vi "Swerve Motor Brushless BL v2.vi"(3 "Offset":dbl, 4 "Drive Commands":T2, 6 "Direction command (deg)":dbl, 7 "Speed command":dbl, 9 "Align 90":bool) -> (0 "Back Left Position":dbl, 1 "Back Left Current Angle":dbl, 2 "Back Left Velocity":dbl)   [LabVIEW 2020]
uses:
  <vilib>/Analysis/coordinate.llb/Angle Units.ctl
  <vilib>/Analysis/coordinate.llb/Angle Range (Degree).ctl
  <vilib>/Rock Robotics/WPI/ThirdParty/REV Robotics/REVLib/Typedef/Spark MAX Control Type.ctl
  <vilib>/Analysis/coordinate.llb/Wrap Angle (scalar).vi
  <vilib>/addons/control/pid/pid.llb/PID (DBL).vi
  <vilib>/Analysis/NI_AAL_Angle.lvlib
  <vilib>/addons/control/pid/NI_PID_pid.lvlib
panel:
  out "Encoder Count to Move":dbl
  out "Better Angle":dbl(knob)=41.7137932364482 scale=0.0..360.0
  out "Degres To Travel":dbl
  out "Position Closed Loop Plots":cluster{"Better Position":dbl, dbl}(graph)
  in  "PID gains":T1={"proportional gain (Kc)"=0.01, "integral time (Ti, min)"=0.0, "derivative time (Td, min)"=0.004} {"integral time (Ti, min)" format="%#_6f"; "derivative time (Td, min)" format="%#_6f"}
  in  "output range":cluster{"output high":dbl, "output low":dbl}={"output high"=0.4, "output low"=-0.4} {"output low" format="%.2f"; "output high" format="%.2f"}
  out "Flip motors?":bool
  out "Better Position":dbl
  # "VI inputs"
  # "Intermediate values"
  # "Click here to set min"
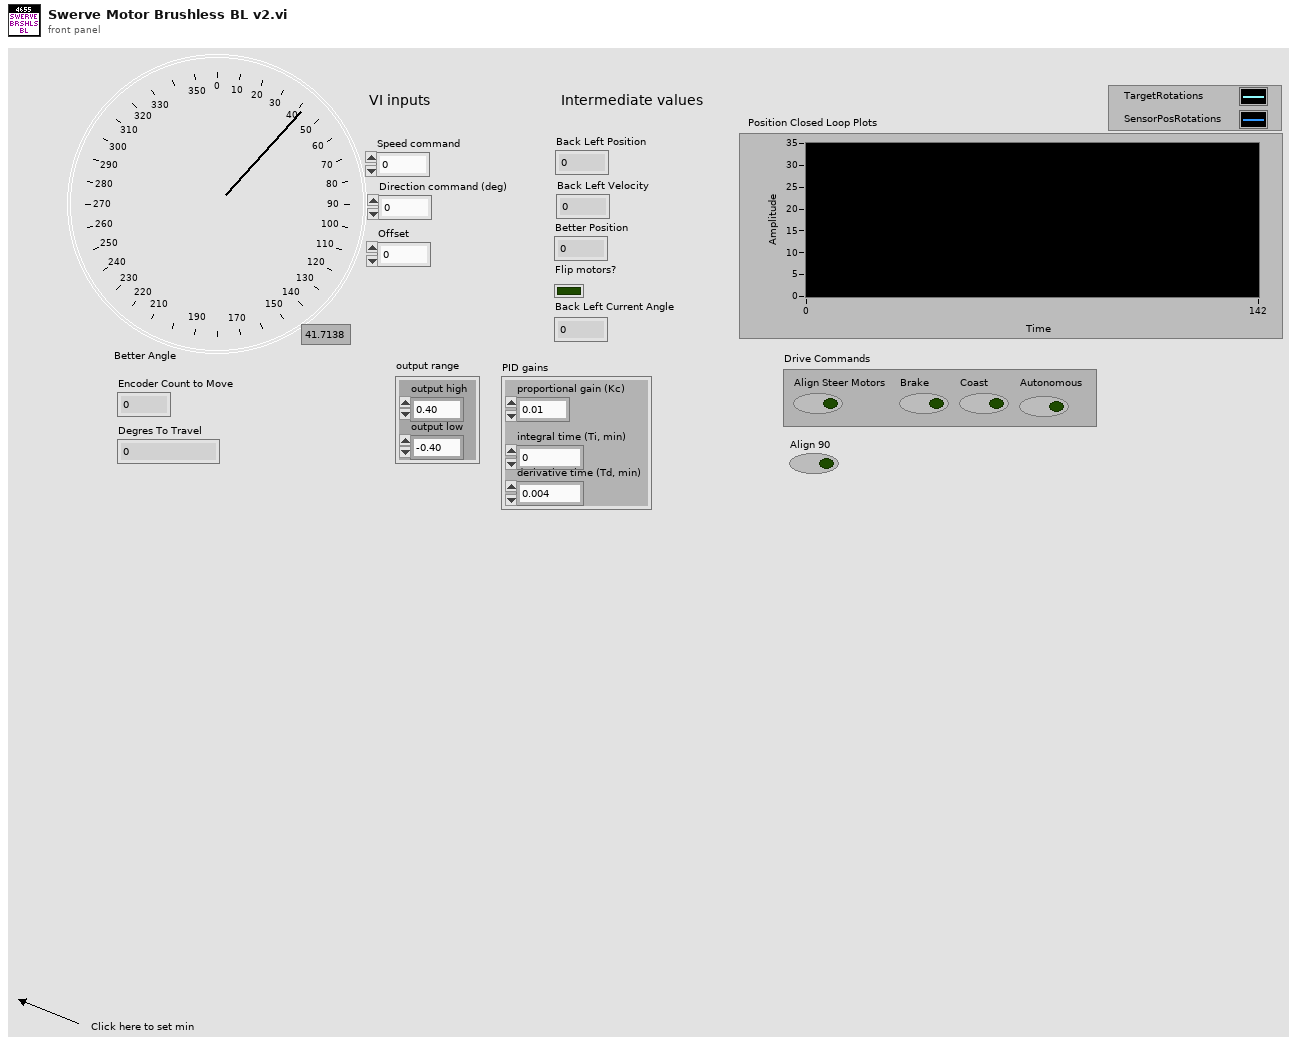
[diagram p1: front panel]
types:
  T1 = cluster{"proportional gain (Kc)":dbl, "integral time (Ti, min)":dbl, "derivative time (Td, min)":dbl}
  T2 = cluster{"Align Steer Motors":bool, "Brake":bool, "Coast":bool, "Autonomous":bool}
  T3 = typedef "NI_AAL_Angle.lvlib/Angle Range (Degree).ctl" = u16
  T4 = typedef "NI_AAL_Angle.lvlib/Angle Units.ctl" = i32
  T5 = typedef "WPI_MotorControlDeviceRef.ctl" = cluster{"DeviceStatus":errorcluster, "Type":T6, "PWM":cluster{"PWM Channel":T7, "DeadBand":T8}, "CAN":cluster{"Device Number":u8, "SetOutput VI Ref":variant, "GetOutput VI Ref":variant, "Enable VI Ref":variant, "Disable VI Ref":variant, "Data":variant}, "Invert":bool, "DIO PWM":cluster{"PWM \"Enable\" Channel":T7, "DIOChannel":T9, "PWM Rate":dbl}}
  T6 = typedef "WPI_MotorControlType.ctl" = enum16{"PWM", "CAN", "DIO PWM"}
  T7 = typedef "FPGA_DIOPWMChannel.ctl" = enum8{"PWM 0", "PWM 1", "PWM 2", "PWM 3", "PWM 4", "PWM 5", "PWM 6", "PWM 7", "PWM 8", "PWM 9", "PWM MXP 0", "PWM MXP 1", "PWM MXP 2", "PWM MXP 3", "PWM MXP 4", "PWM MXP 5", "PWM MXP 6", "PWM MXP 7", "PWM MXP 8", "PWM MXP 9", "Invalid"}
  T8 = typedef "WPI_PWMDeadband.ctl" = cluster{"Name":string, "maxPositivePwm":i32, "minPositivePwm":i32, "centerPwm":i32, "maxNegativePwm":i32, "minNegativePwm":i32, "angularRange":u16}
  T9 = typedef "FPGA_DIOChannel.ctl" = enum8{"DIO 0", "DIO 1", "DIO 2", "DIO 3", "DIO 4", "DIO 5", "DIO 6", "DIO 7", "DIO 8", "DIO 9", "DIO MXP 0", "DIO MXP 1", "DIO MXP 2", "DIO MXP 3", "DIO MXP 4", "DIO MXP 5", "DIO MXP 6", "DIO MXP 7", "DIO MXP 8", "DIO MXP 9", "DIO MXP 10", "DIO MXP 11", "DIO MXP 12", "DIO MXP 13", "DIO MXP 14", "DIO MXP 15", "SPI Port CS1", "SPI Port CS2", "SPI Port CS3", "SPI Port MISO", "SPI Port MOSI", "Invalid"}
  T10 = cluster{"process variable":dbl, "Degres To Travel":dbl}
  T11 = typedef "Spark MAX Control Type.ctl" = enum16{"Percent VBus", "Voltage", "Velocity", "Position", "Smart Motion", "Current", "Smart Velocity"}
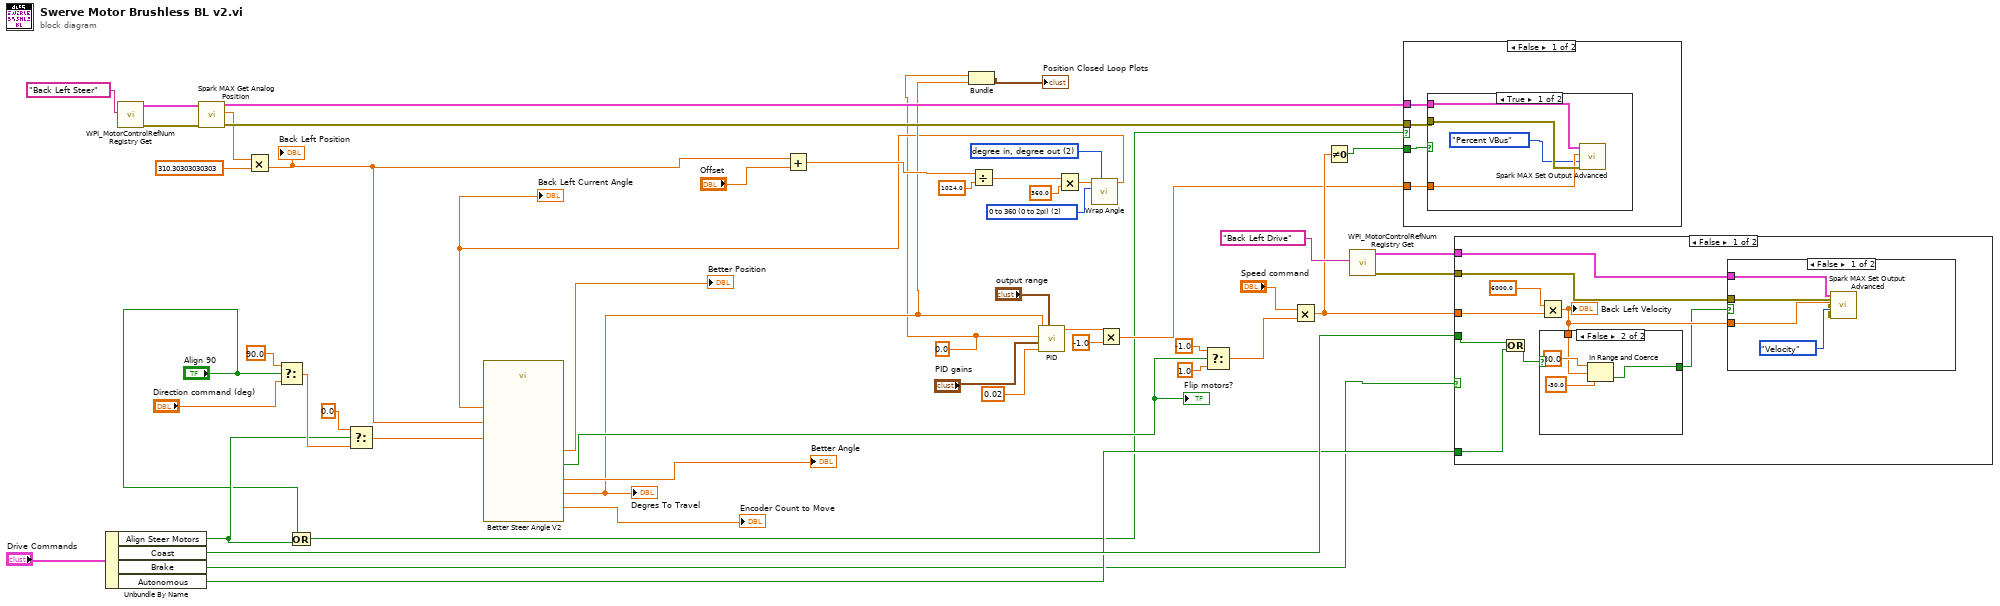
[diagram p0: block diagram]
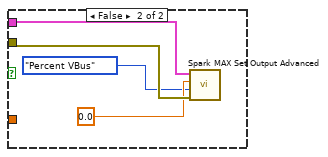
[diagram p2: hidden frame]
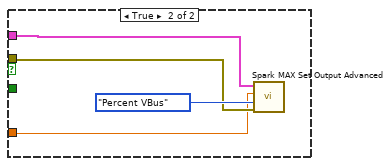
[diagram p3: hidden frame]
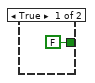
[diagram p4: hidden frame]
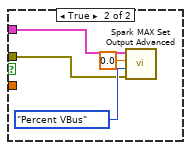
[diagram p5: hidden frame]
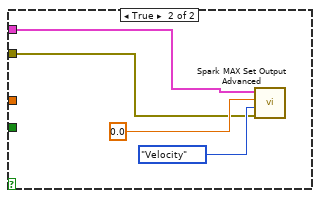
[diagram p6: hidden frame]
diagram:
  w2 = 0.0 ("process variable")
  w42 = T3 2 items=["none", "-180 to 180 (-pi to pi)", "0 to 360 (0 to 2pi)"] ("angle range")
  w43 = T4 2 items=["radian in, radian out", "radian in, degree out", "degree in, degree out", "degree in, radian out"] ("angle units")
  n1 = Unbundle By Name("Drive Commands") -> ("Align Steer Motors"=w10:bool, "Coast"=w38:bool, "Brake"=w36:bool, "Autonomous"=w37:bool)
  n2 = call <vilib>:"WPI_MotorControlRefNum Registry Get.vi"("refnum name"="Back Left Steer" ("Motor References")) -> ("error out"=w34:errorcluster, "RobotDriveDevRef"=w35:T5)  [unwired: 9 in]
  n3 = call <vilib>:"Spark MAX Get Analog Position.vi"("error in (no error)"=w34, "MotorControlDevRef in"=w35) -> ("error out"=w47:errorcluster, "Analog Position"=w18:dbl, "MotorControlDevRef out"=w20:T5)  [unwired: 6 in, 1 out]
  n4 = Multiply(x=w18, y=310.30303030303) -> (x*y=w6:dbl)
  "Back Left Position" <- w6
  n5 = Select(t=90.0, s="Align 90", f="Direction command (deg)") -> (s? t:f=w15:dbl)
  n6 = Or(x="Align 90", y=w10) -> (x .or. y?=w11:bool)
  n7 = Select(t=0.0, s=w10, f=w15) -> (s? t:f=w12:dbl)
  n8 = Add(x=w6, y="Offset") -> (x+y=w23:dbl)
  n9 = Divide(x=w23, y=1024.0 ("x")) -> (x/y=w41:dbl)
  n10 = Multiply(x=w41, y=360.0 ("x*y")) -> (x*y=w40:dbl)
  n11 = call-poly <vilib>:"Wrap Angle.vi"("angle units"=w43, "angle range"=w42, "angle in"=w40) -> ("angle out"=w3:dbl)  [unwired: 7 in, 1 out]
  "Back Left Current Angle" <- w3
  n12 = call "Better Steer Angle V2.vi"("Current Angle"=w3, "Current Position"=w6, "Set Point In"=w12) -> ("Better Angle"=→"Better Angle":dbl, "Better Position"=→"Better Position":dbl, "Encoder Count to Move"=→"Encoder Count to Move":dbl, "Flip motors?"=w46:bool, "Degres To Travel"=w4:dbl)
  "Flip motors?" <- w46
  "Degres To Travel" <- w4
  n13 = Bundle("process variable"=w2, "Degres To Travel"=w4) -> (→"Position Closed Loop Plots":T10)  [unwired: 1 in]
  n14 = call-poly <vilib>:"PID.vi"("output range"="output range", "dt (s)"=0.02, "PID gains"="PID gains", "process variable"=w2, "setpoint"=w4) -> ("output"=w22:dbl)  [unwired: 5 in, 1 out]
  n15 = Multiply(x=w22, y=-1.0) -> (x*y=w19:dbl)
  n16 = Select(t=-1.0, s=w46, f=1.0) -> (s? t:f=w49:dbl)
  n17 = Multiply(x="Speed command", y=w49) -> (x*y=w21:dbl)
  n18 = Not Equal To 0?(x=w21) -> (x != 0?=w1:bool)
  n19 = call <vilib>:"WPI_MotorControlRefNum Registry Get.vi"("refnum name"="Back Left Drive" ("Motor References")) -> ("error out"=w30:errorcluster, "RobotDriveDevRef"=w31:T5)  [unwired: 9 in]
  n20 = case shown="False" w11 {
    tunnel: w47 -> [w55 w66]
    tunnel: w1 -> [w54 _]
    tunnel: w20 -> [w53 w65]
    tunnel: w19 -> [w52 w64]
    frame False {
      n21 = case shown="True" w54 {
        tunnel: w53 -> [w59 w63]
        tunnel: w55 -> [w58 w62]
        tunnel: w52 -> [w57 _]
        frame True {
          n22 = call <vilib>:"Spark MAX Set Output Advanced.vi"("error in (no error)"=w58, "Control Mode"=Spark_MAX_Control_Type."Percent VBus", "Setpoint"=w57, "MotorControlDevRef"=w59) -> ()  [unwired: 6 in, 2 out]
        }
        frame False {
          n23 = call <vilib>:"Spark MAX Set Output Advanced.vi"("error in (no error)"=w62, "Control Mode"=Spark_MAX_Control_Type."Percent VBus", "Setpoint"=0.0 ("y"), "MotorControlDevRef"=w63) -> ()  [unwired: 6 in, 2 out]
        }
      }
    }
    frame True {
      n24 = call <vilib>:"Spark MAX Set Output Advanced.vi"("error in (no error)"=w66, "Control Mode"=Spark_MAX_Control_Type."Percent VBus", "Setpoint"=w64, "MotorControlDevRef"=w65) -> ()  [unwired: 6 in, 2 out]
    }
  }
  n25 = case shown="False" w36 {
    tunnel: w21 -> [w75 _]
    tunnel: w38 -> [w71 _]
    tunnel: w37 -> [w70 _]
    tunnel: w31 -> [w69 w91]
    tunnel: w30 -> [w68 w90]
    frame False {
      n26 = Or(x=w71, y=w70) -> (x .or. y?=w72:bool)
      n27 = Multiply(x=6000.0, y=w75) -> (x*y=w74:dbl)
      "Back Left Velocity" <- w74
      n28 = case shown="False" w72 {
        tunnel: w74 -> [_ w79]
        tunnel: [FALSE w78] -> w73
        frame True {
        }
        frame False {
          n29 = In Range and Coerce(upper limit=30.0, x=w79, lower limit=-30.0) -> (In Range?=w78:bool)  [unwired: 1 out]
        }
      }
      n30 = case shown="False" w73 {
        tunnel: w74 -> [w84 _]
        tunnel: w69 -> [w83 w87]
        tunnel: w68 -> [w82 w86]
        frame False {
          n31 = call <vilib>:"Spark MAX Set Output Advanced.vi"("error in (no error)"=w82, "Control Mode"=Spark_MAX_Control_Type."Velocity", "Setpoint"=w84, "MotorControlDevRef"=w83) -> ()  [unwired: 6 in, 2 out]
        }
        frame True {
          n32 = call <vilib>:"Spark MAX Set Output Advanced.vi"("error in (no error)"=w86, "Control Mode"=Spark_MAX_Control_Type."Percent VBus", "Setpoint"=0.0, "MotorControlDevRef"=w87) -> ()  [unwired: 6 in, 2 out]
        }
      }
    }
    frame True {
      n33 = call <vilib>:"Spark MAX Set Output Advanced.vi"("error in (no error)"=w90, "Control Mode"=Spark_MAX_Control_Type."Velocity", "Setpoint"=0.0, "MotorControlDevRef"=w91) -> ()  [unwired: 6 in, 2 out]
    }
  }
